vi "tune per chan.vi"(10 "channel in":T1, 11 "compensation":T1) -> (2 "channel out":T1)   [LabVIEW 2020]
uses:
  <vilib>/rvi/FXPMathLib/FxpInterpret/XNode/nifxpmath_Interpret.xnode
types:
  T1 = cluster{"Real":fxp<+/-,16,3>, "Imag":fxp<+/-,16,3>}
  T2 = cluster{"Real":fxp<+/-,25,25>, "Imag":fxp<+/-,25,25>}
  T3 = cluster{"Real":fxp<+/-,18,18>, "Imag":fxp<+/-,18,18>}
  T4 = cluster{"Real":fxp<+/-,48,48>, "Imag":fxp<+/-,48,48>}
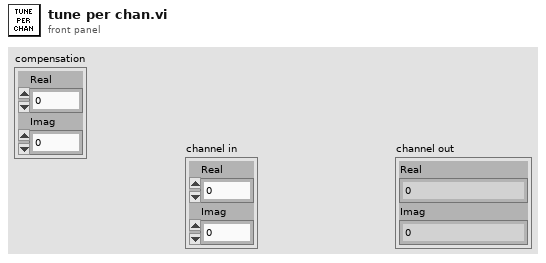
[diagram p1: front panel]
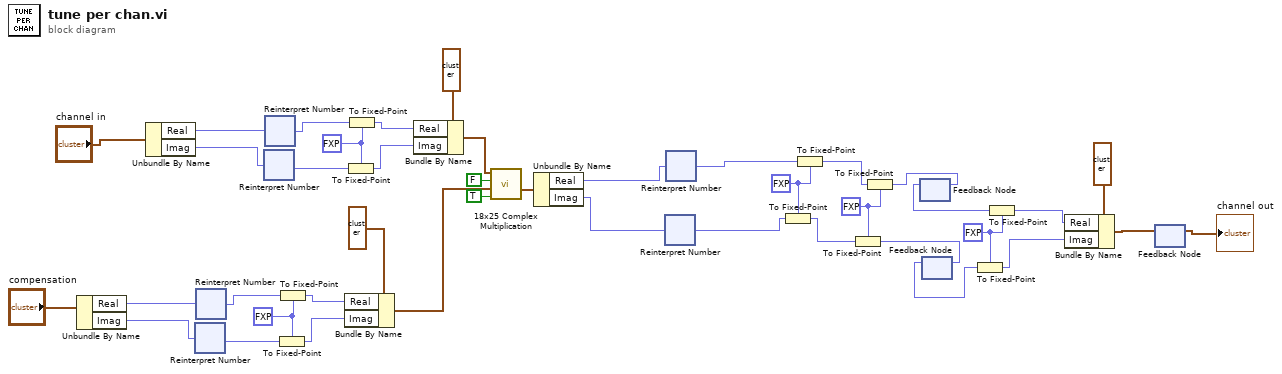
[diagram p0: block diagram]
diagram:
  w14 = fxp<+/-,16,3> 0.0 ("fixed-point type")
  w17 = fxp<+/-,20,7> 0.0 ("fixed-point type")
  w20 = fxp<+/-,42,6> 0.0 ("fixed-point type")
  w27 = fxp<+/-,25,25> 0.0 ("fixed-point type")
  w35 = fxp<+/-,18,18> 0.0 ("fixed-point type")
  n1 = Unbundle By Name("compensation") -> ("Real"=w29:fxp<+/-,16,3>, "Imag"=w28:fxp<+/-,16,3>)
  n2 = Unbundle By Name("channel in") -> ("Real"=w41:fxp<+/-,16,3>, "Imag"=w40:fxp<+/-,16,3>)
  n3 = xnode "Reinterpret Number"("x"=w28) -> ("y"=w23:fxp<+/-,16,16>)
  n4 = xnode "Reinterpret Number"("x"=w29) -> ("y"=w24:fxp<+/-,16,16>)
  n5 = xnode "Reinterpret Number"("x"=w40) -> ("y"=w31:fxp<+/-,16,16>)
  n6 = xnode "Reinterpret Number"("x"=w41) -> ("y"=w32:fxp<+/-,16,16>)
  n7 = To Fixed-Point(fixed-point type=w27, number=w23) -> (fixed-point=w25:fxp<+/-,25,25>)
  n8 = To Fixed-Point(fixed-point type=w27, number=w24) -> (fixed-point=w26:fxp<+/-,25,25>)
  n9 = Bundle By Name(cluster=T2 {"Real"=0.0, "Imag"=0.0} ("Complex"), "Real"=w26, "Imag"=w25) -> (w21:T2)
  n10 = To Fixed-Point(fixed-point type=w35, number=w31) -> (fixed-point=w33:fxp<+/-,18,18>)
  n11 = To Fixed-Point(fixed-point type=w35, number=w32) -> (fixed-point=w34:fxp<+/-,18,18>)
  n12 = Bundle By Name(cluster=T3 {"Real"=0.0, "Imag"=0.0} ("Complex"), "Real"=w34, "Imag"=w33) -> (w38:T3)
  n13 = call "18x25 Complex Multiplication.vi"("conjugate B"=TRUE, "B"=w21, "conjugate A"=FALSE, "A"=w38) -> ("product"=w30:T4)  [unwired: 7 in]
  n14 = Unbundle By Name(w30) -> ("Real"=w5:fxp<+/-,48,48>, "Imag"=w4:fxp<+/-,48,48>)
  n15 = xnode "Reinterpret Number"("x"=w4) -> ("y"=w18:fxp<+/-,48,22>)
  n16 = xnode "Reinterpret Number"("x"=w5) -> ("y"=w19:fxp<+/-,48,22>)
  n17 = To Fixed-Point(fixed-point type=w20, number=w18) -> (fixed-point=w15:fxp<+/-,42,6>)
  n18 = To Fixed-Point(fixed-point type=w20, number=w19) -> (fixed-point=w16:fxp<+/-,42,6>)
  n19 = To Fixed-Point(fixed-point type=w17, number=w15) -> (fixed-point=w11:fxp<+/-,20,7>)
  n20 = To Fixed-Point(fixed-point type=w17, number=w16) -> (fixed-point=w13:fxp<+/-,20,7>)
  n21 = feedback #1() -> (w12:fxp<+/-,20,7>)  [unwired: 1 in]
  n22 = feedback-in #1(w13) -> ()
  n23 = feedback #2() -> (w10:fxp<+/-,20,7>)  [unwired: 1 in]
  n24 = feedback-in #2(w11) -> ()
  n25 = To Fixed-Point(fixed-point type=w14, number=w10) -> (fixed-point=w7:fxp<+/-,16,3>)
  n26 = To Fixed-Point(fixed-point type=w14, number=w12) -> (fixed-point=w8:fxp<+/-,16,3>)
  n27 = Bundle By Name(cluster=T1 {"Real"=0.0, "Imag"=0.0} ("Complex"), "Real"=w8, "Imag"=w7) -> (w6:T1)
  n28 = feedback #3() -> (→"channel out":T1)  [unwired: 1 in]
  n29 = feedback-in #3(w6) -> ()
